vi "DIR RT.vi"(8 "错误输入":errorcluster, 10 "DIR":bool[](array[boolean])=[FALSE, FALSE, FALSE, FALSE, TRUE, TRUE], 11 "Custom FPGA Reference Out":refnum<k20>) -> (0 "错误输出":errorcluster, 3 "FPGA VI引用输出":refnum<k20>)   [LabVIEW 2017]
uses:
  <vilib>/Utility/error.llb/Error Cluster From Error Code.vi
  <vilib>/rvi/errors/niLvFpgaAdjustHostInterfaceError.vi
  <vilib>/rvi/interface/nirviReadWriteControl/nirviReadWriteControl.xnode
  NiFpgaLv.dll
  <vilib>/rvi/interface/Simulation/niFpgaSimulationCallBeginRW.vi
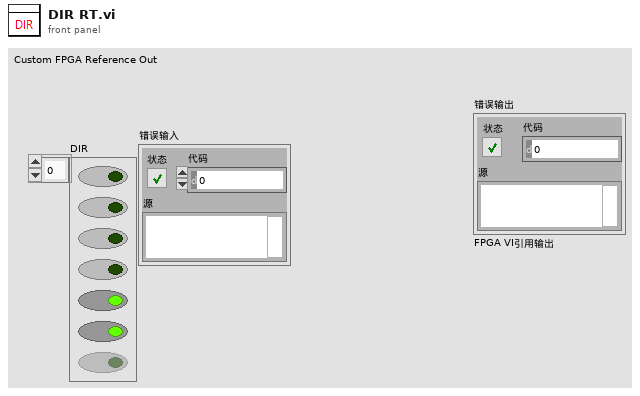
[diagram p1: front panel]
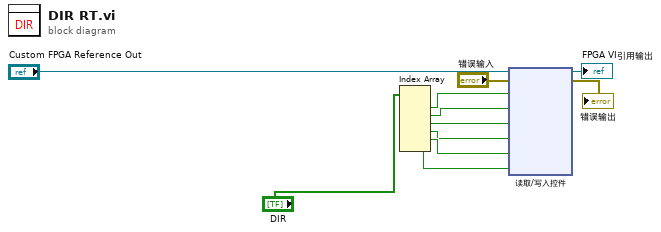
[diagram p0: block diagram]
diagram:
  n1 = Index Array(array="DIR") -> (element #1=w5:bool, element #2=w7:bool, element #3=w8:bool, element #4=w9:bool, element #5=w10:bool, element #6=w11:bool)  [unwired: 6 in]
  n2 = xnode "读取/写入控件"("FPGA VI引用输入"="Custom FPGA Reference Out", "错误输入"="错误输入", "A/DIO5"=w5, "A/DIO6"=w7, "A/DIO7"=w8, "B/DIO7"=w9, "A/DIO4"=w10, "A/DIO13"=w11) -> ("FPGA VI引用输出"=→"FPGA VI引用输出":refnum<k20>, "错误输出"=→"错误输出":errorcluster)
